vi "ACT LG Read Most Recent Logfiles.vi"(0 "Directory Log Path":path, 11 "Error in (no error)":errorcluster) -> (4 "Data":string[][](table), 15 "Error out":errorcluster)   [LabVIEW 2011]
doc: "This VI is used for the purpose of logging data to a file. The \"Directory Log Name\" should contain the directory name that you want your log files to be placed. This directory MUST have a \"_\" (i.e., \"underscore\") contained in it. An example would be: BEESON_DIR. The VI checks to see if your directory is valid and then will name all of your logfiles \"BEESON_[n].log\" were \"n\" is a U32 integer pertaining to the order in which the file was created. A new logfile will dynamically be created based on the current logfile's size in comparison to the \"Size Limit.\" The most recent logfile will always be filled to capacity before the next one is created.\n\nIf files are deleted from the logfile directory in use then the vi will create a file next in the sequence of previously used numbers.\n\nThis scheme of logging data will support 4,294,967,295 files per directory, and at 250k a piece will top out at around 1,000 Tera-Bytes Maximum--well beyond any PCs capabilities! So delete old files before your disk becomes full.\n\nThis vi was created by David Gianetto, contact me with any problems, questions, etc."
uses:
  File IO/Type Defs/FILE Type Enum.ctl
panel:
  in  "Files to Read (2)":i32=2
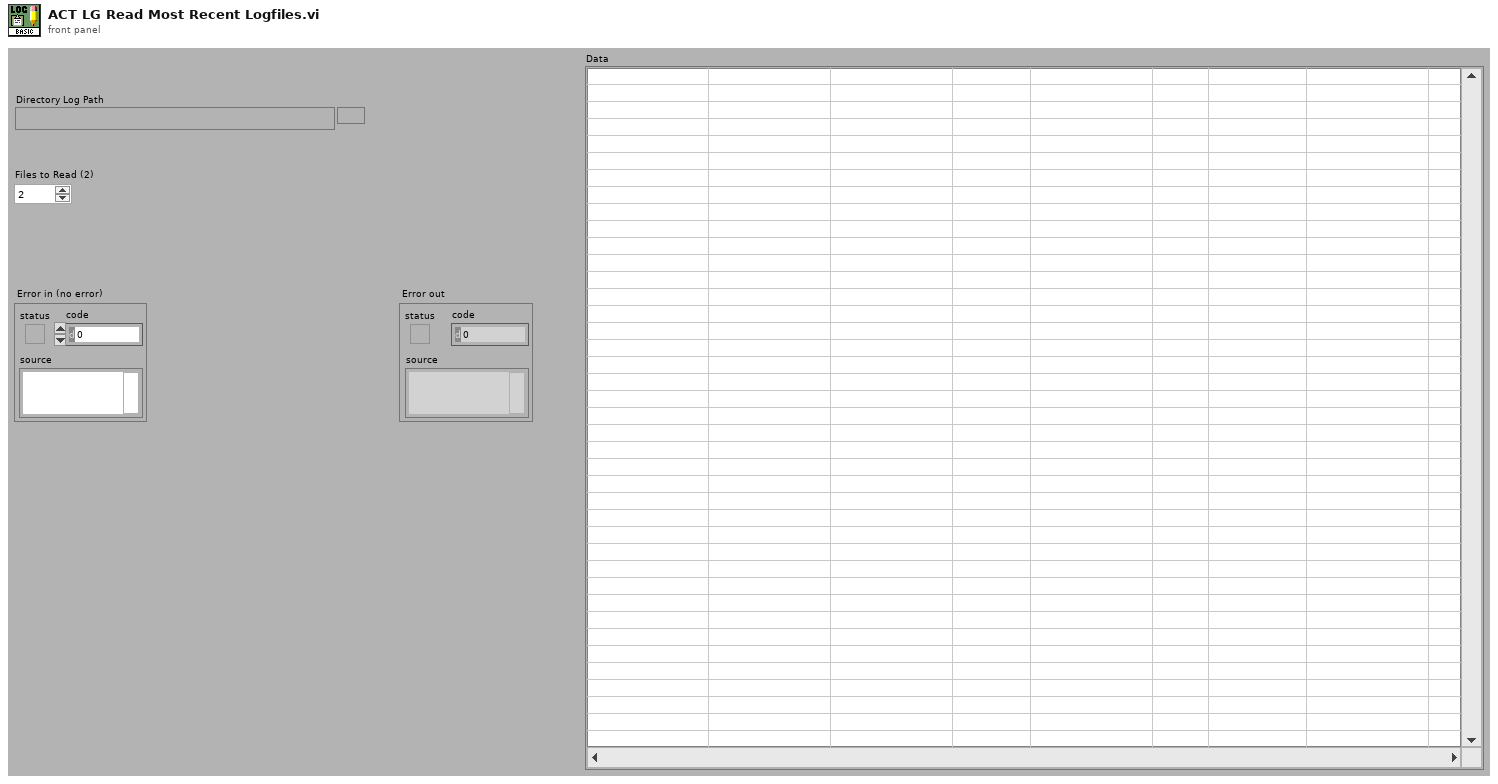
[diagram p1: front panel]
types:
  T1 = typedef "FILE Type Enum.ctl" = enum16{"Text", "Spreadsheet"}
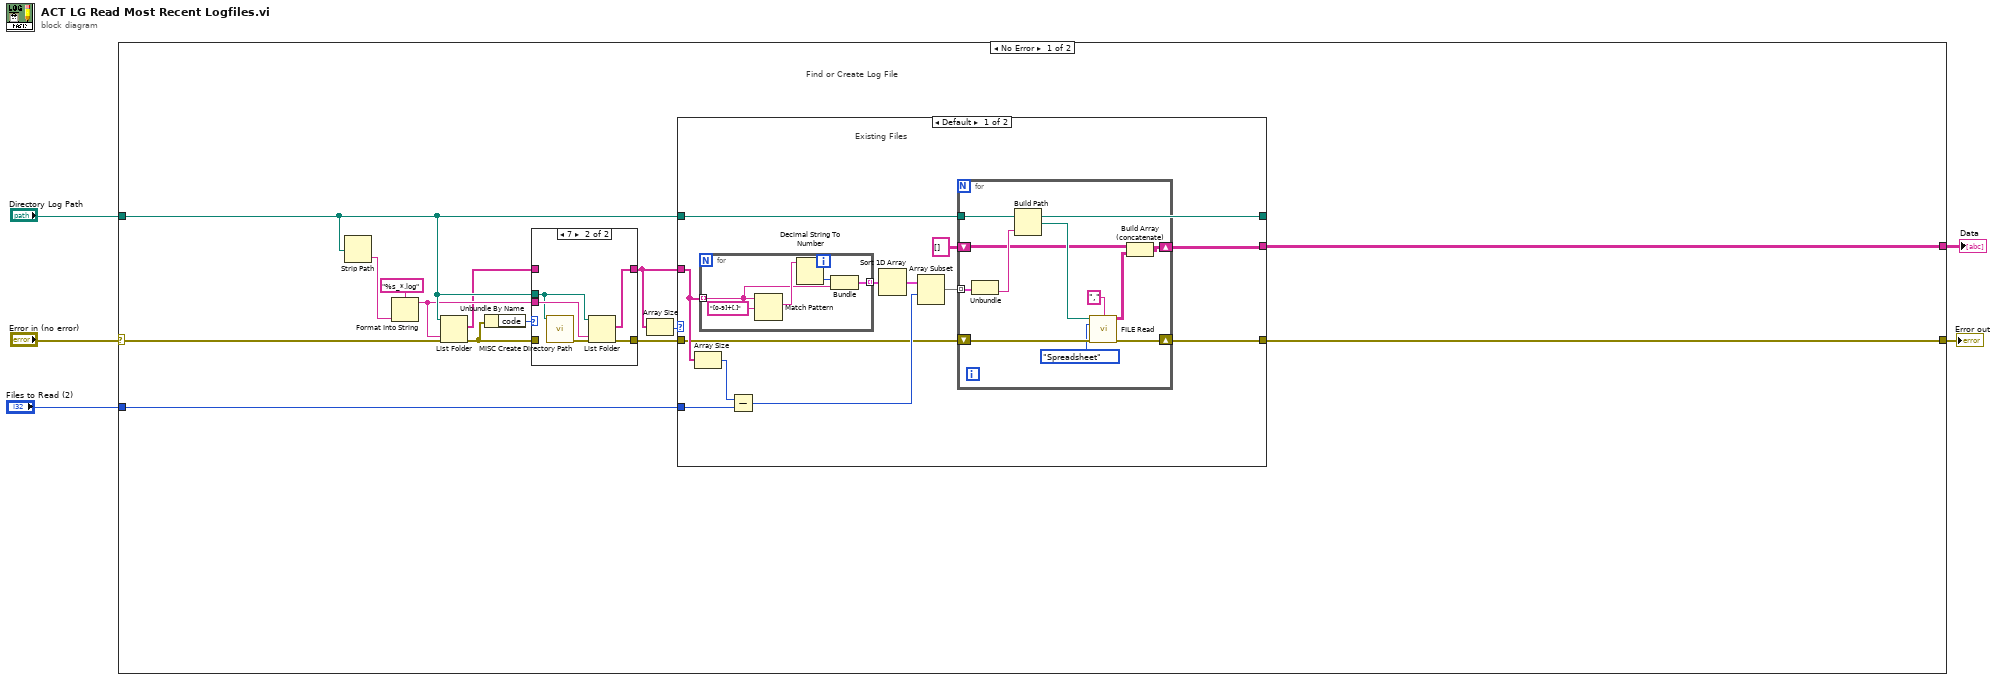
[diagram p0: block diagram]
diagram:
  n1 = case shown="No Error" "Error in (no error)" {
    selector: "Error in (no error)" -> [w18 w57]
    tunnel: "Directory Log Path" -> [w19 _]
    tunnel: [w8 w57] -> w5
    tunnel: "Files to Read (2)" -> [w7 _]
    tunnel: [w6 _] -> w1
    frame No Error {
      # "Find or Create Log File"
      n2 = Strip Path(path=w19) -> (name=w17:string)  [unwired: 1 out]
      n3 = Format Into String(format string="%s_*.log", w17) -> (resulting string=w11:string)  [unwired: 2 in, 1 out]
      n4 = List Folder(path=w19, pattern=w11, error in=w18) -> (filenames=w10:string[], error out=w12:errorcluster)  [unwired: 3 out]
      n5 = Unbundle By Name(w12) -> ("code"=w13:i32)
      n6 = case shown="7" w13 {
        tunnel: [w21 w25] -> w14
        tunnel: w12 -> [w21 _]
        tunnel: w19 -> [_ w22]
        tunnel: w11 -> [_ w24]
        tunnel: [w20 w23] -> w9
        tunnel: w10 -> [w20 _]
        frame Default {
        }
        frame 7 {
          n7 = call "MISC Create Directory Path.vi"("Path"=w22) -> ("Error Out"=w26:errorcluster)  [unwired: 2 in, 12 out]
          n8 = List Folder(path=w22, pattern=w24, error in=w26) -> (filenames=w23:string[], error out=w25:errorcluster)  [unwired: 3 out]
        }
      }
      n9 = Array Size(array=w9) -> (size(s)=w15:i32)
      n10 = case shown="Default" w15 {
        tunnel: w9 -> [w35 _]
        tunnel: [w29 w56] -> w8
        tunnel: w19 -> [w38 w55]
        tunnel: w14 -> [w30 w56]
        tunnel: [w38 w55] -> _
        tunnel: w7 -> [w33 _]
        tunnel: [w27 _] -> w6
        frame Default {
          # "Existing Files"
          n11 = Array Size(array=w35) -> (size(s)=w34:i32)
          n12 = for {
            tunnel: w35 -> [w51] mode=indexing
            tunnel: [w50] -> w37 mode=indexing
            n13 = Match Pattern(string=w51, regular expression="[0-9]+[.]") -> (match substring=w53:string)  [unwired: 4 out]
            n14 = Decimal String To Number(string=w53) -> (number=w52:i32)  [unwired: 3 out]
            n15 = Bundle(w52, w51) -> (w50:cluster{i32, string})  [unwired: 1 out]
          }
          n16 = Subtract(x=w34, y=w33) -> (x-y=w32:i32)
          n17 = Sort 1D Array(array=w37) -> (sorted array=w36:cluster{i32, string}[])
          n18 = Array Subset(array=w36, index=w32) -> (w31:cluster{i32, string}[])  [unwired: 1 in]
          n19 = for {
            tunnel: w38 -> [w49]
            tunnel: w31 -> [w48] mode=indexing
            shift-right: [w44] -> w29
            shift-left: w30 -> [w45]
            shift-right: [w40] -> w27
            shift-left: string[][] [] -> [w39]
            n20 = Unbundle(w48) -> (w47:string)  [unwired: 1 out]
            n21 = Build Path(base path=w49, name or relative path=w47) -> (appended path=w46:path)
            n22 = call "FILE Read.vi"("File Path (dialog if empty)"=w46, "Delimiter (Tab)"=",", "File Type (text)"=FILE_Type_Enum."Spreadsheet", "Error In (no error)"=w45) -> ("Spreadsheet Data (all)"=w41:string[][], "Error Out"=w44:errorcluster)  [unwired: 3 in, 7 out]
            n23 = Build Array (concatenate)(w39, w41) -> (w40:string[][])
          }
        }
        frame 0 {
          # "No Existing Files"
        }
      }
    }
    frame Error {
    }
  }
  "Error out" <- w5
  "Data" <- w1
